vi "sub_solver_algorithm.vi"(10 "# iterations w/o changes":i32, 11 "status":enum16{"unsolved", "solved", "invalid state"}(ring)) -> (2 "solved ?":bool, 3 "commands":string[](array[string]))   [LabVIEW 2018]
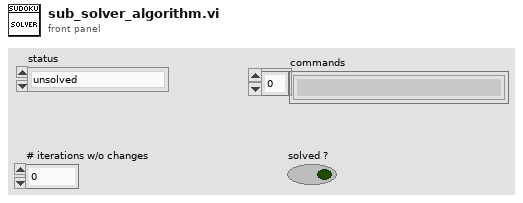
[diagram p1: front panel]
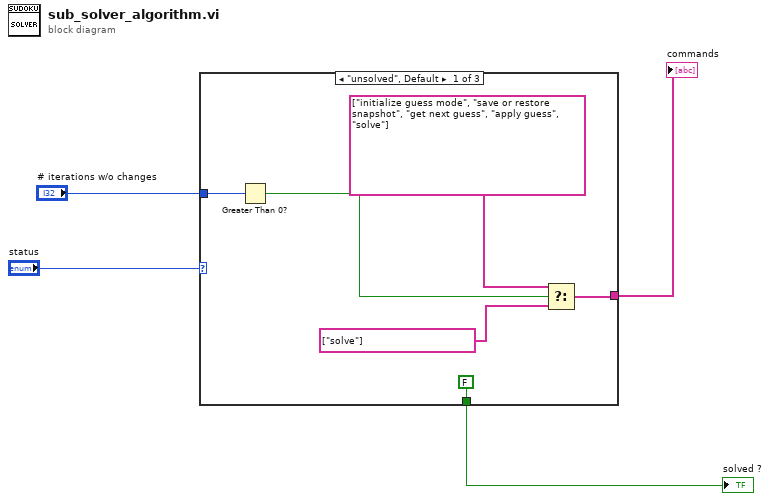
[diagram p0: block diagram]
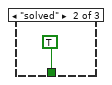
[diagram p2: hidden frame]
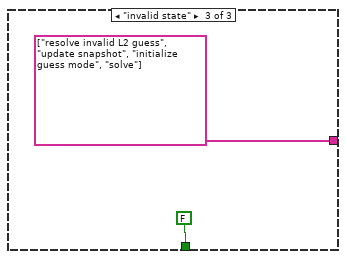
[diagram p3: hidden frame]
diagram:
  n1 = case shown="\"unsolved\", Default" "status" {
    tunnel: [FALSE TRUE FALSE] -> w2
    tunnel: "# iterations w/o changes" -> [w5 _ _]
    tunnel: [w6 _ string[] ["resolve invalid L2 guess", "update snapshot", "initialize guess mode", "solve"] ("commands")] -> w4
    frame "unsolved", Default {
      n2 = Greater Than 0?(x=w5) -> (x > 0?=w9:bool)
      n3 = Select(t=string[] ["initialize guess mode", "save or restore snapshot", "get next guess", "apply guess", "solve"] ("commands"), s=w9, f=string[] ["solve"] ("commands")) -> (s? t:f=w6:string[])
    }
    frame "solved" {
    }
    frame "invalid state" {
    }
  }
  "commands" <- w4
  "solved ?" <- w2
